vi "Network.vi"() -> (0 "dB refl":dbl format="%#_3g", 1 "V Pwr":dbl format="%#_4g", 2 "deg refl":dbl format="%_3g", 3 "V phase":dbl format="%#_4g")   [LabVIEW 2013]
panel:
  out "Write Array 6":i32[](array[numeric])
  out "Read Array 6":i32[](array[numeric])
  out "Bytes Read 6":i32
  out "Bytes Written 6":i32
  out "Bytes Written 5":i32
  out "Bytes Read 5":i32
  out "Read Array 5":i32[](array[numeric])
  out "Write Array 5":i32[](array[numeric])
  out "ADC word 3":i32
  out "Bytes Written 4":i32
  out "Bytes Read 4":i32
  out "Read Array 4":i32[](array[numeric])
  out "Write Array 4":i32[](array[numeric])
  out "ADC word 2":i32
  out "V Ref":dbl format="%#_4g"
  out "ADC word":i32
  out "Write Array 3":i32[](array[numeric])
  out "Read Array 3":i32[](array[numeric])
  out "Bytes Read 3":i32
  out "Bytes Written 3":i32
  out "Write Array 2":i32[](array[numeric])
  out "Read Array 2":i32[](array[numeric])
  out "Bytes Read 2":i32
  out "Bytes Written 2":i32
  # "AD8302 Readback"
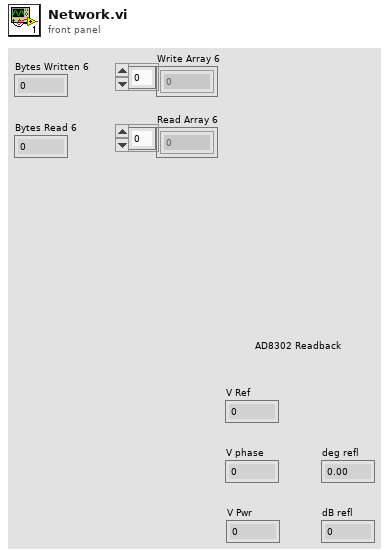
[diagram p1: front panel]
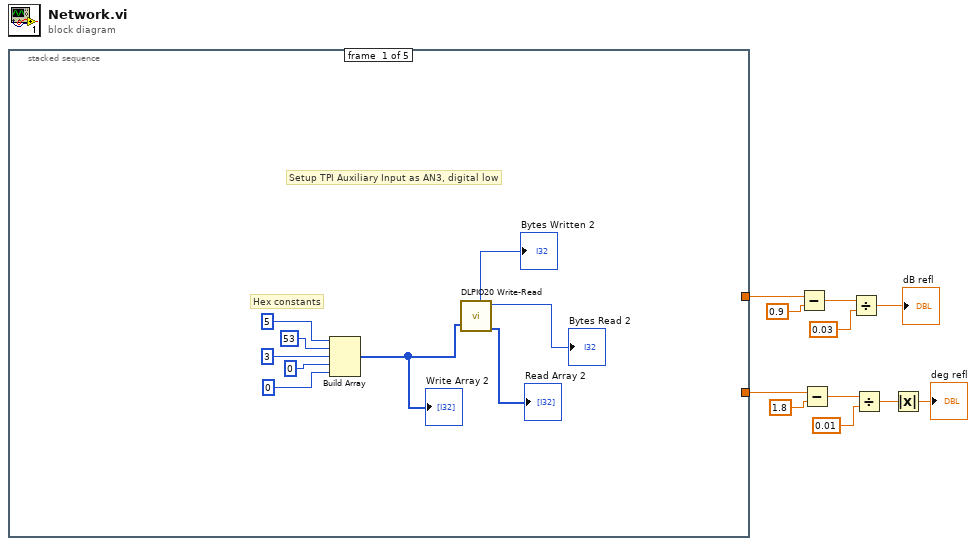
[diagram p0: block diagram]
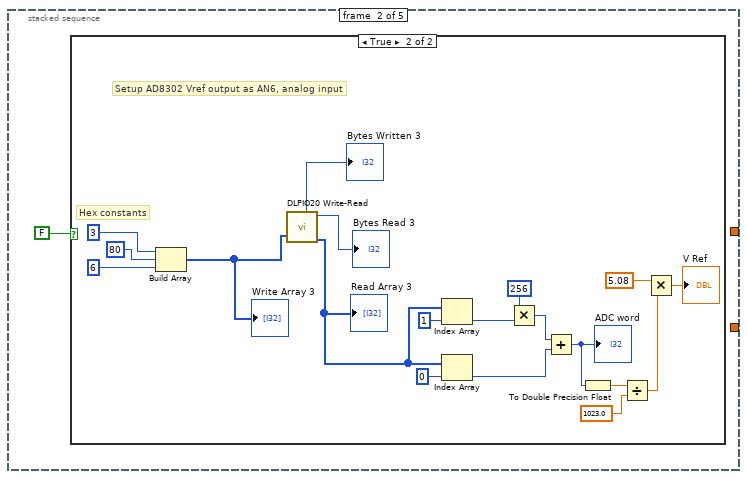
[diagram p2: hidden frame]
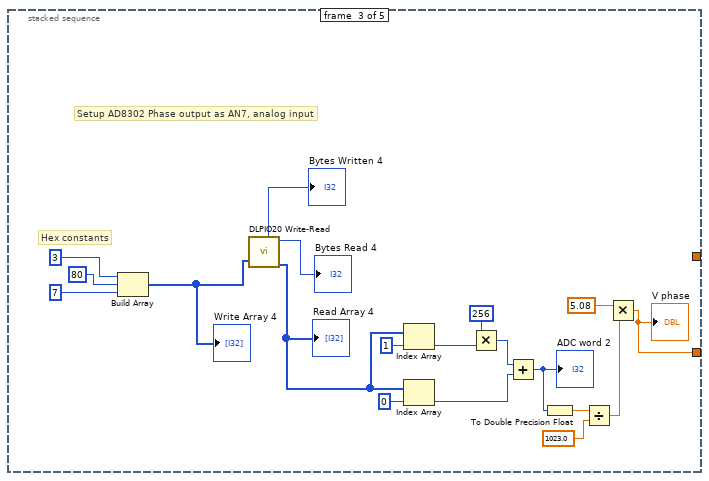
[diagram p4: hidden frame]
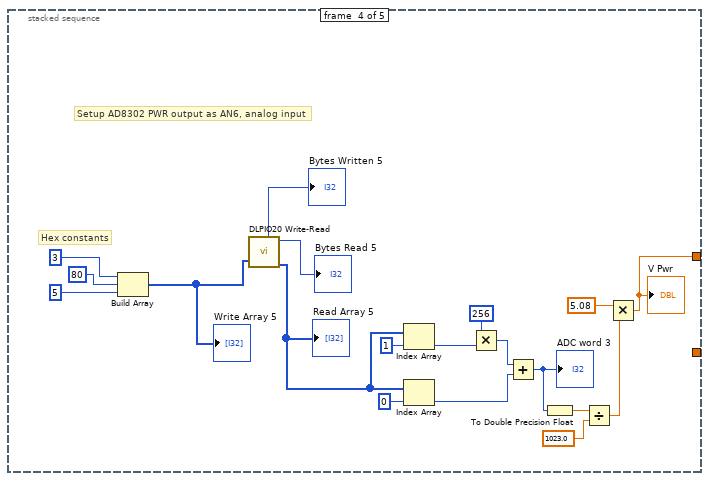
[diagram p5: hidden frame]
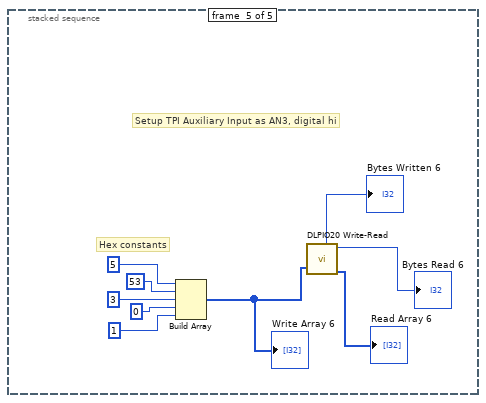
[diagram p6: hidden frame]
diagram:
  n1 = stacked-sequence {
    tunnel: [_ _ w41 _ _] -> w3
    tunnel: [_ _ _ w60 _] -> w11
    frame #0 {
      # "Setup TPI Auxiliary Input as AN3, digital low"
      # "Hex constants"
      n2 = Build Array "Build Array"(u8 5, u8 53, u8 3, u8 0, u8 0) -> (w15:u8[])
      "Write Array 2" <- w15
      n3 = call "DLPIO20 Write-Read.vi"("Write Buffer"=w15) -> ("Read Buffer Out"=→"Read Array 2":u8[], "Bytes Read"=→"Bytes Read 2":u32, "Bytes Written"=→"Bytes Written 2":u32)  [unwired: 3 in]
    }
    frame #1 {
      n4 = case shown="True" FALSE {
        frame False {
        }
        frame True {
          # "Setup AD8302 Vref output as AN6, analog input"
          # "Hex constants"
          n5 = Build Array "Build Array"(u8 3, u8 80, u8 6) -> (w36:u8[])
          "Write Array 3" <- w36
          n6 = call "DLPIO20 Write-Read.vi"("Write Buffer"=w36) -> ("Read Buffer Out"=w34:u8[], "Bytes Read"=→"Bytes Read 3":u32, "Bytes Written"=→"Bytes Written 3":u32)  [unwired: 3 in]
          "Read Array 3" <- w34
          n7 = Index Array "Index Array"(array=w34, index=1) -> (element=w31:u8)
          n8 = Index Array(array=w34, index=0) -> (element=w28:u8)
          n9 = Multiply(x=256, y=w31) -> (x*y=w29:i32)
          n10 = Add(x=w29, y=w28) -> (x+y=w27:i32)
          "ADC word" <- w27
          n11 = To Double Precision Float(number=w27) -> (double precision float=w26:dbl)
          n12 = Divide(x=w26, y=1023.0) -> (x/y=w23:dbl)
          n13 = Multiply(x=5.08, y=w23) -> (x*y=→"V Ref":dbl)
        }
      }
    }
    frame #2 {
      # "Setup AD8302 Phase output as AN7, analog input"
      # "Hex constants"
      n14 = Build Array "Build Array"(u8 3, u8 80, u8 7) -> (w55:u8[])
      "Write Array 4" <- w55
      n15 = call "DLPIO20 Write-Read.vi"("Write Buffer"=w55) -> ("Read Buffer Out"=w53:u8[], "Bytes Read"=→"Bytes Read 4":u32, "Bytes Written"=→"Bytes Written 4":u32)  [unwired: 3 in]
      "Read Array 4" <- w53
      n16 = Index Array "Index Array"(array=w53, index=1) -> (element=w50:u8)
      n17 = Index Array(array=w53, index=0) -> (element=w47:u8)
      n18 = Multiply(x=256, y=w50) -> (x*y=w48:i32)
      n19 = Add(x=w48, y=w47) -> (x+y=w46:i32)
      "ADC word 2" <- w46
      n20 = To Double Precision Float(number=w46) -> (double precision float=w45:dbl)
      n21 = Divide(x=w45, y=1023.0) -> (x/y=w42:dbl)
      n22 = Multiply(x=5.08, y=w42) -> (x*y=w41:dbl)
      "V phase" <- w41
    }
    frame #3 {
      # "Setup AD8302 PWR output as AN6, analog input"
      # "Hex constants"
      n23 = Build Array "Build Array"(u8 3, u8 80, u8 5) -> (w74:u8[])
      "Write Array 5" <- w74
      n24 = call "DLPIO20 Write-Read.vi"("Write Buffer"=w74) -> ("Read Buffer Out"=w72:u8[], "Bytes Read"=→"Bytes Read 5":u32, "Bytes Written"=→"Bytes Written 5":u32)  [unwired: 3 in]
      "Read Array 5" <- w72
      n25 = Index Array "Index Array"(array=w72, index=1) -> (element=w69:u8)
      n26 = Index Array(array=w72, index=0) -> (element=w66:u8)
      n27 = Multiply(x=256, y=w69) -> (x*y=w67:i32)
      n28 = Add(x=w67, y=w66) -> (x+y=w65:i32)
      "ADC word 3" <- w65
      n29 = To Double Precision Float(number=w65) -> (double precision float=w64:dbl)
      n30 = Divide(x=w64, y=1023.0) -> (x/y=w61:dbl)
      n31 = Multiply(x=5.08, y=w61) -> (x*y=w60:dbl)
      "V Pwr" <- w60
    }
    frame #4 {
      # "Setup TPI Auxiliary Input as AN3, digital hi"
      # "Hex constants"
      n32 = Build Array "Build Array"(u8 5, u8 53, u8 3, u8 0, u8 1) -> (w82:u8[])
      "Write Array 6" <- w82
      n33 = call "DLPIO20 Write-Read.vi"("Write Buffer"=w82) -> ("Read Buffer Out"=→"Read Array 6":u8[], "Bytes Read"=→"Bytes Read 6":u32, "Bytes Written"=→"Bytes Written 6":u32)  [unwired: 3 in]
    }
  }
  n34 = Subtract(x=w11, y=0.9) -> (x-y=w9:dbl)
  n35 = Subtract(x=w3, y=1.8) -> (x-y=w5:dbl)
  n36 = Divide(x=w9, y=0.03) -> (x/y=→"dB refl":dbl)
  n37 = Divide(x=w5, y=0.01) -> (x/y=w2:dbl)
  n38 = Absolute Value(x=w2) -> (abs(x)=→"deg refl":dbl)
